vi "CONEX-LDS Get Current Configuration Parameters v2.vi"(11 "Connection Cluster in":T1) -> (1 "Configuration parameters":string, 3 "Connection Cluster out":T1)   [LabVIEW 2010]
doc: "ZT - Get current configuration parameters\n\nOutput:\n - Current configuration parameters"
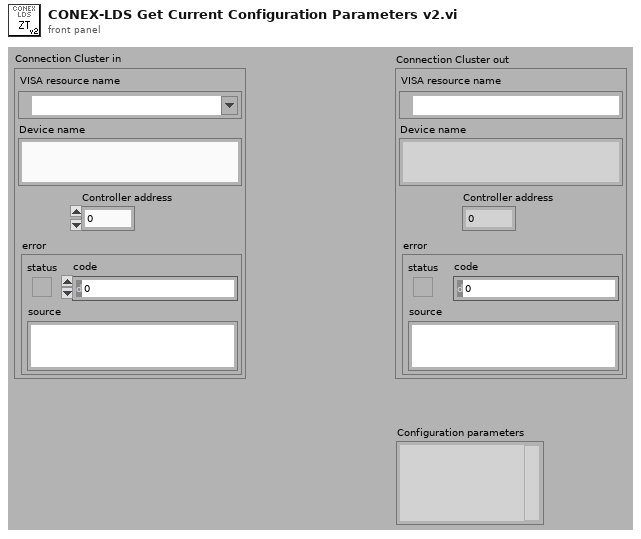
[diagram p1: front panel]
types:
  T1 = cluster{"VISA resource name":refnum<visa-resource-name>, "Device name":string, "Controller address":i32, "error":errorcluster}
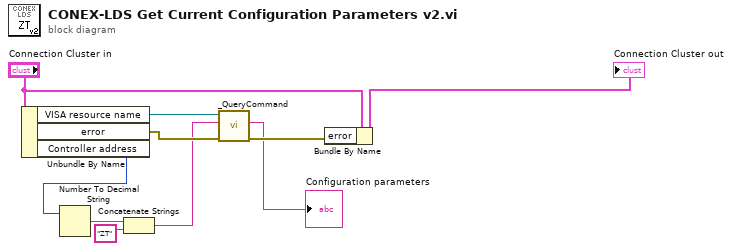
[diagram p0: block diagram]
diagram:
  n1 = Unbundle By Name("Connection Cluster in") -> ("VISA resource name"=w4:refnum<visa-resource-name>, "error"=w8:errorcluster, "Controller address"=w1:i32)
  n2 = Number To Decimal String(number=w1) -> (decimal integer string=w10:string)  [unwired: 1 out]
  n3 = Concatenate Strings(w10, "ZT" ("strCommand")) -> (w3:string)
  n4 = call <userlib>:"_QueryCommand.vi"("error in"=w8, "Command"=w3, "Instrument Channel in"=w4) -> ("error out"=w6:errorcluster, "Response"=→"Configuration parameters":string)  [unwired: 6 in, 1 out]
  n5 = Bundle By Name(cluster="Connection Cluster in", "error"=w6) -> (→"Connection Cluster out":T1)
